vi "Page Channel.vi"(8 "error in (no error)":errorcluster, 11 "Node Ptr":T1 format="%.0x") -> (0 "error out":errorcluster)   [LabVIEW 2017, in "PXImc System Explorer.lvlib"]
uses:
  PXImc System Explorer.lvlib
  <vilib>/NI Veristand/Custom Device API/Custom Device Item Ref.ctl
  <vilib>/NI Veristand/Custom Device API/Custom Device Channel Type.ctl
  <vilib>/NI VeriStand/Custom Device API/Custom Device API.lvlib
panel:
  in  "Default Value":dbl
  out "Channel Settings":i32(listbox)
  in  "Header":cluster{"Section Name":string}={"Section Name"="PXImc Channel Settings"}
  in  "Description":string
  in  "Name":string
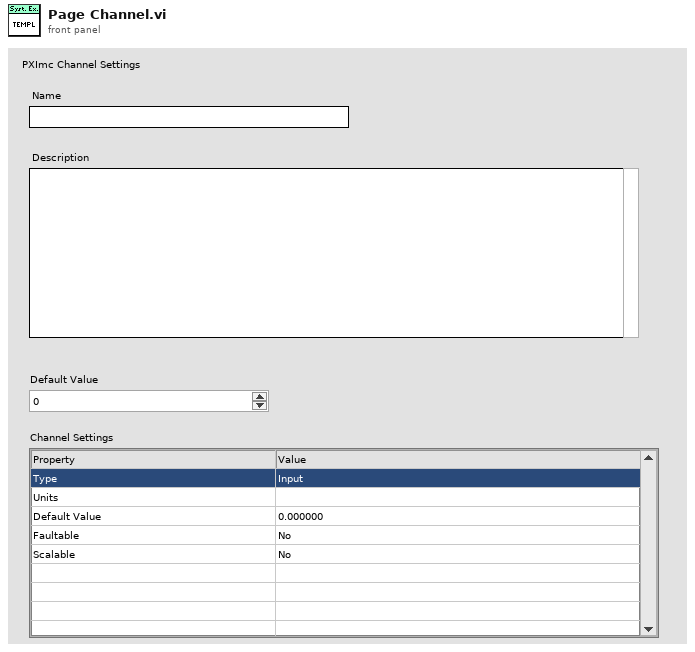
[diagram p1: front panel]
types:
  T1 = typedef "Custom Device API.lvlib/Custom Device Item Ref.ctl" = u64
  T2 = typedef "Custom Device API.lvlib/Custom Device Channel Type.ctl" = enum16{"Input", "Output"}
  T3 = typedef "Custom Device API.lvlib/Custom Device Channel.ctl" = cluster{"Type":T2, "Units":string, "Default Value":dbl, "Faultable":bool, "Scalable":bool}
  T4 = typedef "Custom Device API.lvlib/Custom Device Item Info.ctl" = cluster{"Name":string, "Is Channel":bool, "GUID":string, "Is Waveform":bool}
  T5 = typedef "Custom Device API.lvlib/Custom Device Commands.ctl" = enum16{"Default", "Item renamed", "Shutdown", "Dynamic button pressed"}
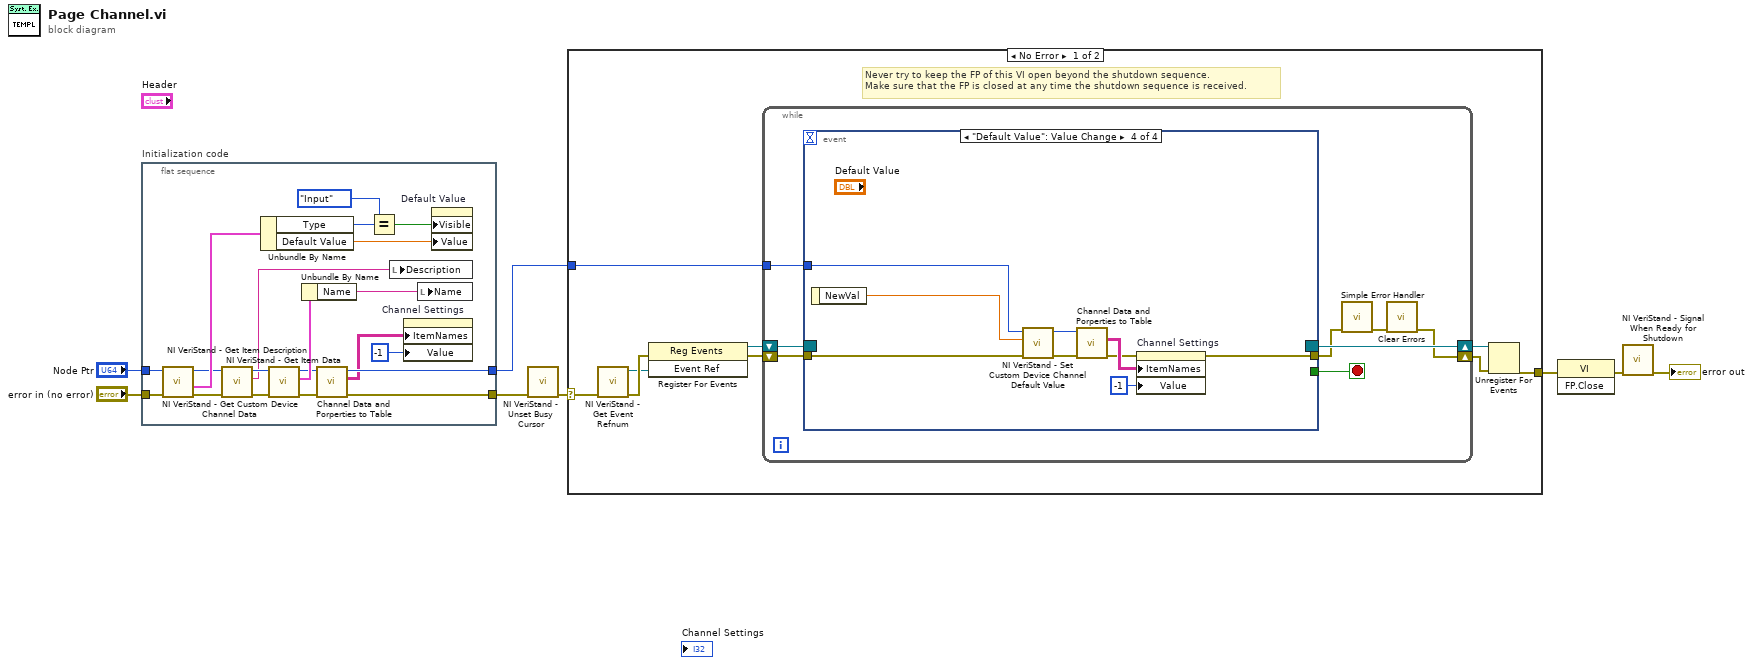
[diagram p0: block diagram]
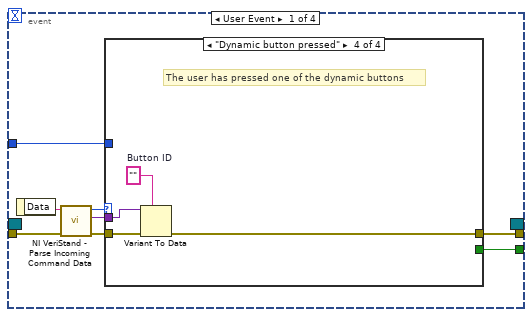
[diagram p2: hidden frame]
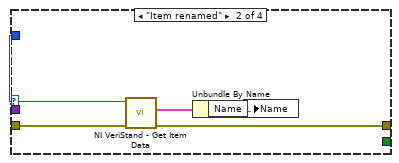
[diagram p4: hidden frame]
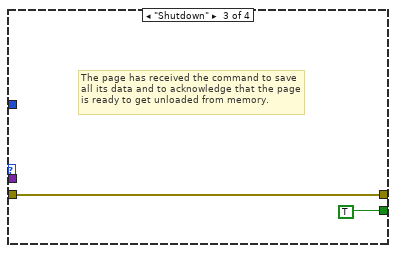
[diagram p5: hidden frame]
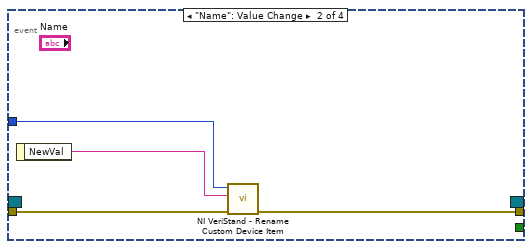
[diagram p6: hidden frame]
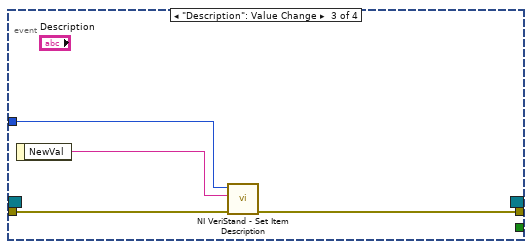
[diagram p7: hidden frame]
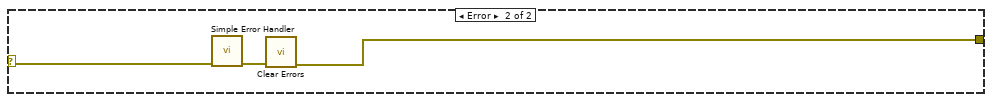
[diagram p8: hidden frame]
diagram:
  n1 = flat-sequence "Initialization code" {
    tunnel: "error in (no error)" -> [w14]
    tunnel: "Node Ptr" -> [w15]
    tunnel: [w21] -> w5
    tunnel: [w22] -> w2
    frame #0 {
      n2 = call <vilib>:"NI VeriStand - Get Custom Device Channel Data.vi"("error in (no error)"=w14, "Channel Ref in"=w15) -> ("error out"=w13:errorcluster, "Channel"=w19:T3, "Channel Ref out"=w16:T1)  [unwired: 4 in, 3 out]
      n3 = call <vilib>:"NI VeriStand - Get Item Description.vi"("error in (no error)"=w13, "Item Ref in"=w16) -> ("error out"=w26:errorcluster, "Description"=w27:string, "Item Ref out"=w28:T1)  [unwired: 7 out]
      n4 = Unbundle By Name(w19) -> ("Type"=w12:T2, "Default Value"=w10:dbl)
      n5 = call <vilib>:"NI VeriStand - Get Item Data.vi"("error in (no error)"=w26, "Item Ref in"=w28) -> ("error out"=w17:errorcluster, "Item Info"=w25:T4, "Item Ref out"=w18:T1)  [unwired: 7 out]
      n6 = Unbundle By Name(w25) -> ("Name"=w24:string)
      n7 = call "Channel Data and Porperties to Table.vi"("error in (no error)"=w17, "Node Ptr"=w18) -> ("error out"=w21:errorcluster, "Properties List Out"=w20:string[][], "Channel Ref out"=w22:T1)  [unwired: 7 in]
      n8 = Equal?(x=Custom_Device_Channel_Type."Input" ("Type"), y=w12) -> (x = y?=w9:bool)
      n9 = local write "Description"(w27) -> ()
      n10 = property on="Channel Settings" class="MCListbox (strict)"("ItemNames"=w20, "Value"=-1 ("Channel Settings")) -> ()  [unwired: 2 in, 2 out]
      n11 = local write "Name"(w24) -> ()
      n12 = property on="Default Value" class="DigNum (strict)"("Visible"=w9, "Value"=w10) -> ()  [unwired: 2 in, 2 out]
    }
  }
  n13 = call <vilib>:"NI VeriStand - Unset Busy Cursor.vi"("error in (no error)"=w5) -> ("error out"=w4:errorcluster)  [unwired: 10 out]
  n14 = case shown="No Error" w4 {
    selector: w4 -> [w29 w85]
    tunnel: [w34 w83] -> w8
    tunnel: w2 -> [w30 _]
    frame No Error {
      # "Never try to keep the FP of this VI open beyond the shutdown sequence.\nMake sure that the FP is closed at any time the shutdown sequence is received."
      n15 = call <vilib>:"NI VeriStand - Get Event Refnum.vi"("error in (no error)"=w29) -> ("error out"=w37:errorcluster, "Event Ref"=w33:refnum<user-event>)  [unwired: 9 out]
      n16 = register-events(error in=w37, w33) -> (reference out=w31:refnum<event-registration>, error out=w32:errorcluster)  [unwired: 1 in]
      n17 = while {
        tunnel: w30 -> [w41]
        shift-right: [w38] -> w35
        shift-left: w32 -> [w44]
        shift-right: [w45] -> w36
        shift-left: w31 -> [w43]
        stop <- w42 stop-if-true
        n18 = event shown="[3] \"Default Value\": Value Change" {
          selector: w43 -> [_ _ _ _]
          dyn-events: [_ _ _ _] -> w45
          timeout: _ -> [_ _ _ _]
          tunnel: w44 -> [w53 w69 w72 w80]
          tunnel: [w49 _ _ _] -> w42
          tunnel: [w48 w68 w71 w74] -> w40
          tunnel: w41 -> [w47 w67 w73 w81]
          event User Event {
            n19 = event-data() -> ("Data"=w52:string)  [unwired: 1 out]
            n20 = call <vilib>:"NI VeriStand - Parse Incoming Command Data.vi"("error in (no error)"=w53, "Incoming data"=w52) -> ("error out"=w51:errorcluster, "Outgoing data"=w46:variant, "Action"=w50:T5)  [unwired: 7 out]
            n21 = case shown="\"Dynamic button pressed\"" w50 {
              tunnel: w51 -> [w54 w59 w60 w65]
              tunnel: [_ _ TRUE _] -> w49
              tunnel: [w54 w56 w60 w62] -> w48
              tunnel: w47 -> [_ w58 _ _]
              tunnel: w46 -> [_ _ _ w64]
              frame "Default", Default {
              }
              frame "Item renamed" {
                n22 = call <vilib>:"NI VeriStand - Get Item Data.vi"("error in (no error)"=w59, "Item Ref in"=w58) -> ("error out"=w56:errorcluster, "Item Info"=w57:T4)  [unwired: 8 out]
                n23 = Unbundle By Name(w57) -> ("Name"=w55:string)
                n24 = local write "Name"(w55) -> ()
              }
              frame "Shutdown" {
                # "The page has received the command to save all its data and to acknowledge that the page is ready to get unloaded from memory."
              }
              frame "Dynamic button pressed" {
                w63 = ""  # Button ID
                # "The user has pressed one of the dynamic buttons"
                n25 = Variant To Data(error in=w65, type=w63, Variant=w64) -> (error out=w62:errorcluster)  [unwired: 1 out]
              }
            }
          }
          event "Name": Value Change {
            n26 = event-data() -> ("NewVal"=w66:string)  [unwired: 1 out]
            n27 = call <vilib>:"NI VeriStand - Rename Custom Device Item.vi"("error in (no error)"=w69, "New Name"=w66, "Item Ref in"=w67) -> ("error out"=w68:errorcluster)  [unwired: 1 in, 7 out]
          }
          event "Description": Value Change {
            n28 = event-data() -> ("NewVal"=w70:string)  [unwired: 1 out]
            n29 = call <vilib>:"NI VeriStand - Set Item Description.vi"("error in (no error)"=w72, "Description"=w70, "Item Ref in"=w73) -> ("error out"=w71:errorcluster)  [unwired: 8 out]
          }
          event "Default Value": Value Change {
            n30 = event-data() -> ("NewVal"=w82:dbl)  [unwired: 1 out]
            n31 = call <vilib>:"NI VeriStand - Set Custom Device Channel Default Value.vi"("error in (no error)"=w80, "Default Value"=w82, "Channel Ref in"=w81) -> ("error out"=w77:errorcluster, "Channel Ref out"=w76:T1)  [unwired: 7 in]
            n32 = call "Channel Data and Porperties to Table.vi"("error in (no error)"=w77, "Node Ptr"=w76) -> ("error out"=w75:errorcluster, "Properties List Out"=w79:string[][])  [unwired: 7 in, 1 out]
            n33 = property on="Channel Settings" class="MCListbox (strict)"(error in=w75, "ItemNames"=w79, "Value"=-1 ("Channel Settings")) -> (error out=w74:errorcluster)  [unwired: 1 in, 1 out]
          }
        }
        n34 = call <vilib>:"Simple Error Handler.vi"("error in (no error)"=w40) -> ("error out"=w39:errorcluster)  [unwired: 1 in, 7 out]
        n35 = call <vilib>:"Clear Errors.vi"("error in (no error)"=w39) -> ("error out"=w38:errorcluster)  [unwired: 1 in, 5 out]
      }
      n36 = Unregister For Events(event registration refnum=w36, error in=w35) -> (error out=w34:errorcluster)
    }
    frame Error {
      n37 = call <vilib>:"Simple Error Handler.vi"("error in (no error)"=w85) -> ("error out"=w84:errorcluster)  [unwired: 1 in, 7 out]
      n38 = call <vilib>:"Clear Errors.vi"("error in (no error)"=w84) -> ("error out"=w83:errorcluster)  [unwired: 1 in, 5 out]
    }
  }
  n39 = invoke class="VI" method="FP.Close"(error in=w8) -> (error out=w7:errorcluster)  [unwired: 2 in, 2 out]
  n40 = call <vilib>:"NI VeriStand - Signal When Ready for Shutdown.vi"("error in (no error)"=w7) -> ("error out"=→"error out":errorcluster)  [unwired: 10 out]
